vi "Find Next Timestamp.vi"(8 "error in (no error)":errorcluster, 11 "Weekly in":refnum<class "Weekly.lvclass">) -> (0 "error out":errorcluster, 3 "Weekly out":refnum<class "Weekly.lvclass">)   [LabVIEW 2020, in "Weekly.lvclass"]
uses:
  Weekly.lvclass
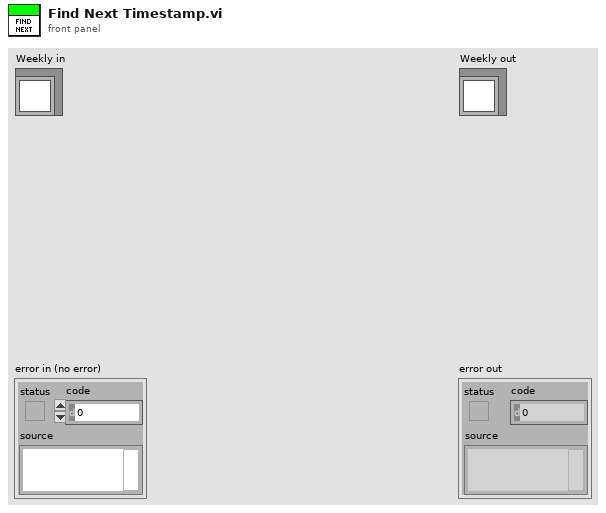
[diagram p1: front panel]
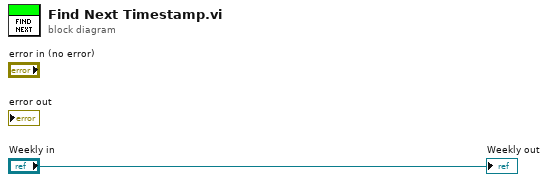
[diagram p0: block diagram]
diagram:
  "Weekly out" <- "Weekly in"
